vi "MID_IR_CM_to_NEAR_IR_NM.vi"(11 "MID IR / cm-1":dbl) -> (3 "Near IR / nm":dbl format="%#_6f")   [LabVIEW 2020]
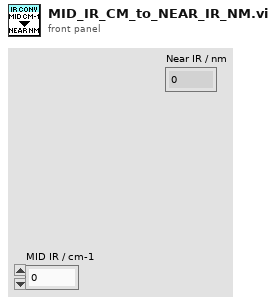
[diagram p1: front panel]
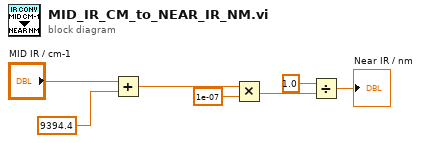
[diagram p0: block diagram]
diagram:
  n1 = Add(x="MID IR / cm-1", y=9394.4) -> (x+y=w5:dbl)
  n2 = Multiply(x=w5, y=1e-07) -> (x*y=w3:dbl)
  n3 = Divide(x=1.0, y=w3) -> (x/y=→"Near IR / nm":dbl)
